vi "RTS Station Save Settings.vi"(8 "Error In":errorcluster, 10 "Data":T1={"Clients"=[], "Listener"=refnum, "Data Array"=["1-1 PF C:\\Technology Lab\\NI-2010\\Trunk\\Refrigeration\\RTS\\Old System\\Point\\16P00290.Pnt"]}, 11 "RTS Config Setup Input":T2) -> (0 "Error Out":errorcluster, 3 "RTS Config Setup Output":T2)   [LabVIEW 2016]
uses:
  Type Definitions/RTS Configuration Setup.ctl
  Type Definitions/RTS Wago Config.ctl
  Type Definitions/RTS APLUS Config.ctl
  Type Definitions/RTS Yokogawa MX Config.ctl
  Type Definitions/RTS Replay Server Control.ctl
  Type Definitions/RTS Server Configuration.ctl
  Type Definitions/RTS Station Settions TCP Comms.ctl
  Type Definitions/RTS Chamber Save Status.ctl
  Type Definitions/RTS Test Pattern.ctl
  Type Definitions/RTS TCP Multiple Connections Data.ctl
  <vilib>/Utility/error.llb/whitespace.ctl
  Type Definitions/RTS TCP Commands.ctl
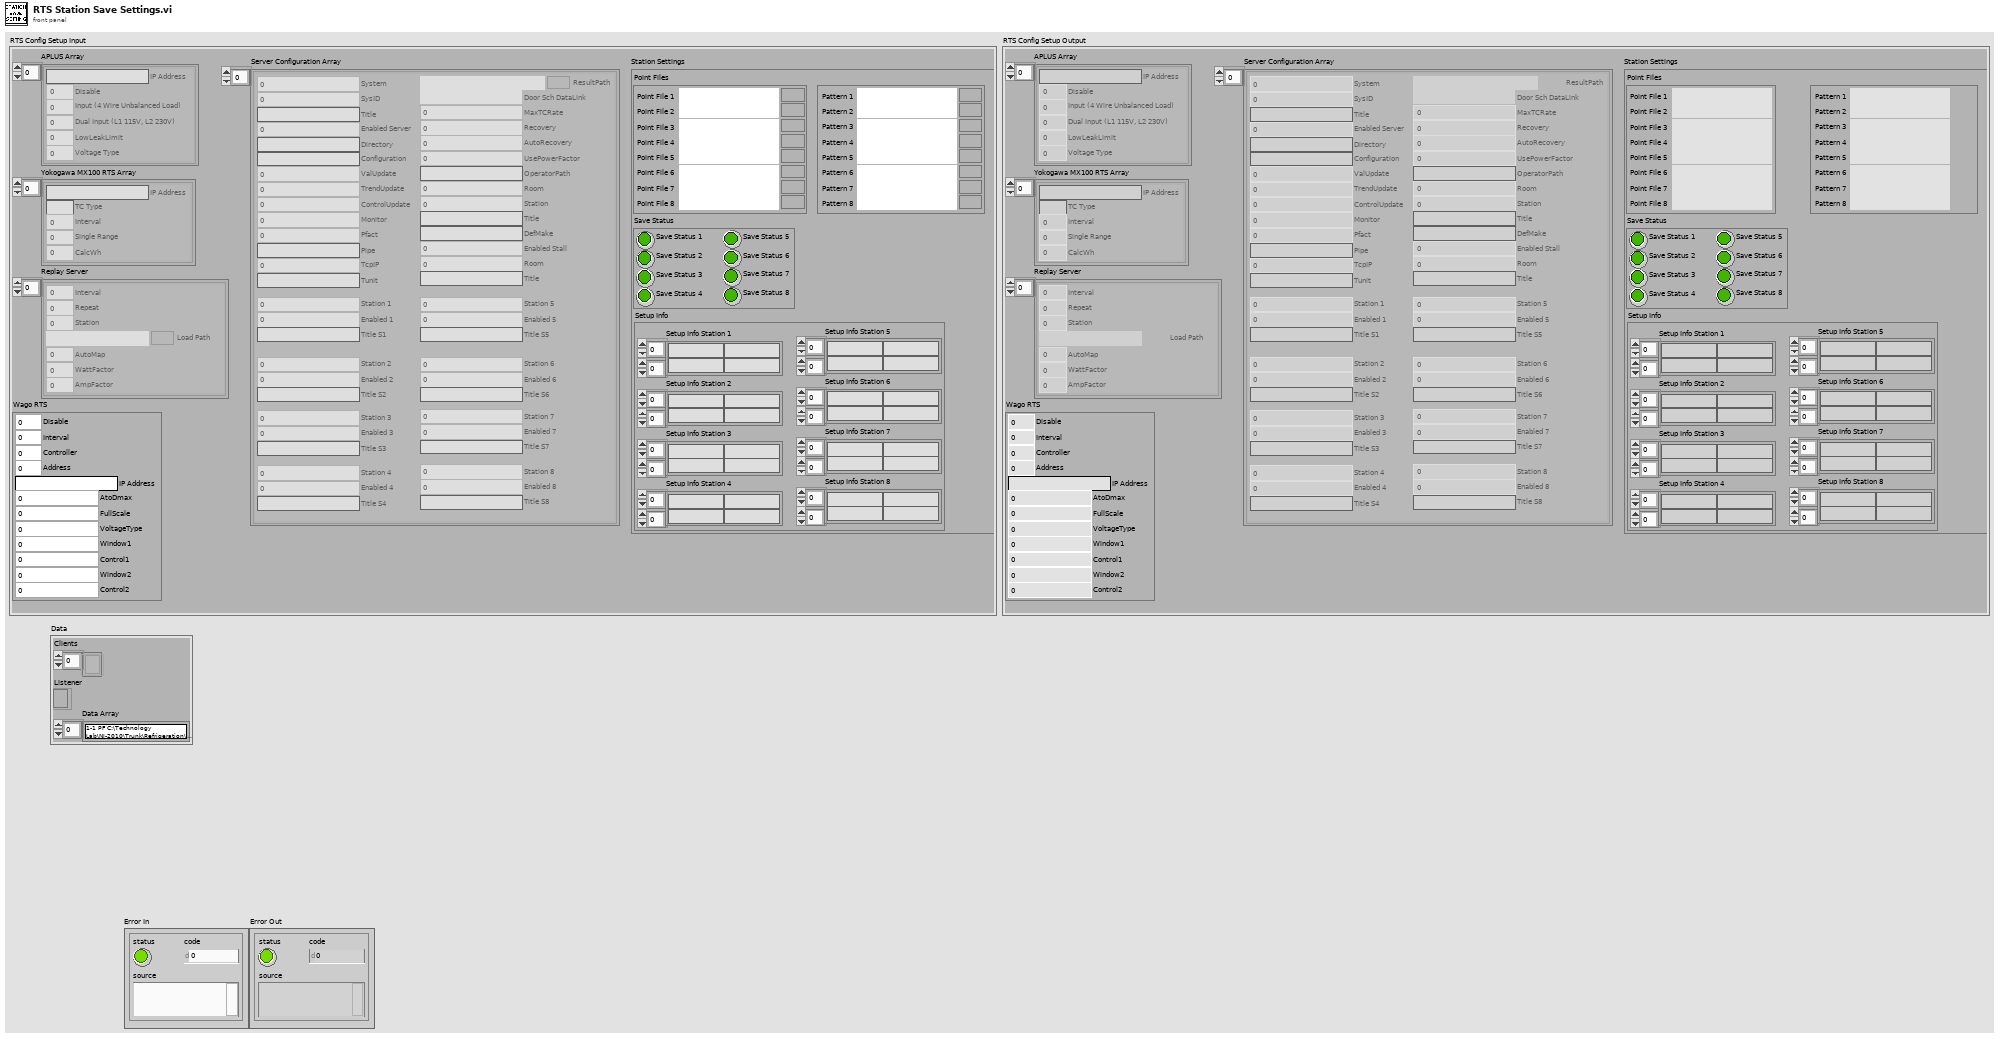
[diagram p1: front panel]
types:
  T1 = typedef "RTS TCP Multiple Connections Data.ctl" = cluster{"Clients":refnum<k5>[], "Listener":refnum<k5>, "Data Array":string[]}
  T2 = typedef "RTS Configuration Setup.ctl" = cluster{"Wago RTS":T3, "APLUS Array":T4[], "Yokogawa MX100 RTS Array":T5[], "Replay Server":T6[], "Server Configuration Array":T7[], "Station Settings":T8}
  T3 = typedef "RTS Wago Config.ctl" = cluster{"Disable":u16, "Interval":u16, "Controller":u16, "Address":u16, "IP Address":string, "AtoDmax":u16, "FullScale":u16, "VoltageType":u16, "Window1":u16, "Control1":u16, "Window2":u16, "Control2":u16}
  T4 = typedef "RTS APLUS Config.ctl" = cluster{"Disable":u16, "IP Address":string, "Input (4 Wire Unbalanced Load)":u16, "Dual Input (L1 115V, L2 230V)":u16, "LowLeakLimit":dbl, "Voltage Type":u16}
  T5 = typedef "RTS Yokogawa MX Config.ctl" = cluster{"IP Address":string, "TC Type":string, "Interval":u16, "Single Range":u16, "CalcWh":u16}
  T6 = typedef "RTS Replay Server Control.ctl" = cluster{"Interval":i16, "Repeat":u16, "Station":u16, "Load Path":path, "AutoMap":u16, "WattFactor":dbl, "AmpFactor":dbl}
  T7 = typedef "RTS Server Configuration.ctl" = cluster{"System":u16, "SysID":u16, "Title":string, "Enabled Server":u16, "Directory":string, "Configuration":string, "ValUpdate":u16, "TrendUpdate":u16, "ControlUpdate":u16, "Monitor":u16, "Pfact":u16, "Pipe":string, "TcpIP":u16, "Tunit":string, "ResultPath":path, "Door Sch DataLink":path, "MaxTCRate":u16, "Recovery":u16, "AutoRecovery":u16, "UsePowerFactor":u16, "OperatorPath":string, "Room":u16, "Station":u16, "Title":string, "DefMake":string, "Enabled Stall":u16, "Room":u16, "Title":string, "Station 1":u16, "Enabled 1":u16, "Station 2":u16, "Enabled 2":u16, "Station 3":u16, "Enabled 3":u16, "Station 4":u16, "Enabled 4":u16, "Station 5":u16, "Enabled 5":u16, "Station 6":u16, "Enabled 6":u16, "Station 7":u16, "Enabled 7":u16, "Station 8":u16, "Enabled 8":u16, "Title S1":string, "Title S2":string, "Title S3":string, "Title S5":string, "Title S6":string, "Title S7":string, "Title S8":string, "Title S4":string}
  T8 = typedef "RTS Station Settions TCP Comms.ctl" = cluster{"Point Files":cluster{"Point File 1":path, "Point File 2":path, "Point File 3":path, "Point File 4":path, "Point File 5":path, "Point File 6":path, "Point File 7":path, "Point File 8":path}, "Save Status":T9, "Setup Info":cluster{"Setup Info Station 1":string[][], "Setup Info Station 2":string[][], "Setup Info Station 3":string[][], "Setup Info Station 4":string[][], "Setup Info Station 5":string[][], "Setup Info Station 6":string[][], "Setup Info Station 7":string[][], "Setup Info Station 8":string[][]}, "Chamber Test Pattern":T10}
  T9 = typedef "RTS Chamber Save Status.ctl" = cluster{"Save Status 1":bool, "Save Status 2":bool, "Save Status 3":bool, "Save Status 4":bool, "Save Status 5":bool, "Save Status 6":bool, "Save Status 7":bool, "Save Status 8":bool}
  T10 = typedef "RTS Test Pattern.ctl" = cluster{" Pattern 1":path, "Pattern 2":path, "Pattern 3":path, "Pattern 4":path, "Pattern 5":path, "Pattern 6":path, "Pattern 7":path, "Pattern 8":path}
  T11 = typedef "RTS TCP Commands.ctl" = string
  T12 = typedef "whitespace.ctl" = u16
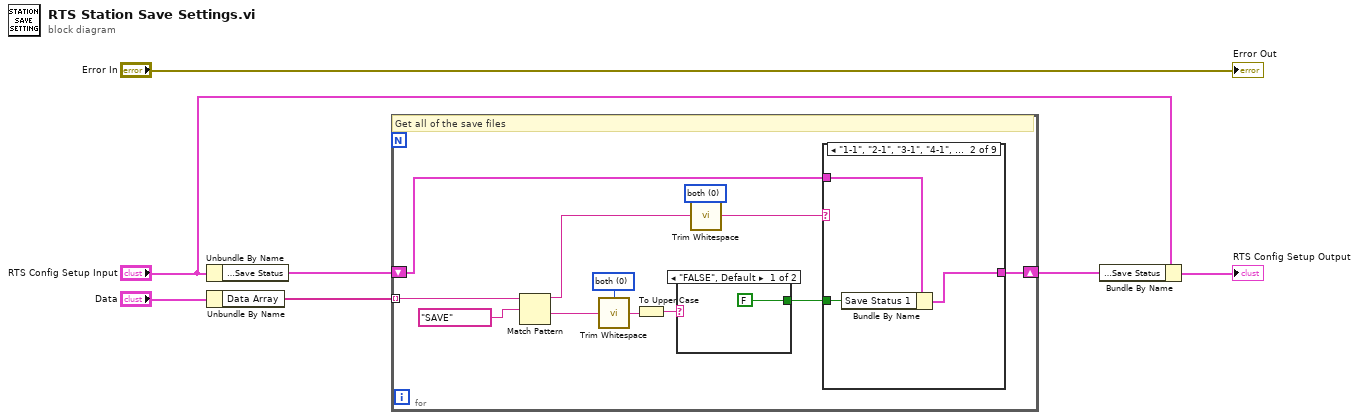
[diagram p0: block diagram]
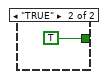
[diagram p2: hidden frame]
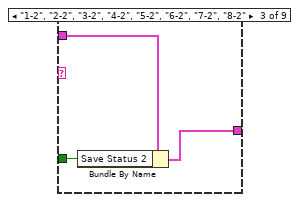
[diagram p4: hidden frame]
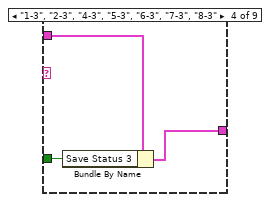
[diagram p5: hidden frame]
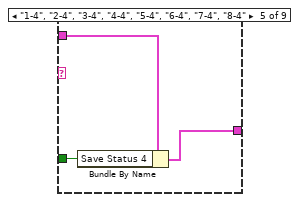
[diagram p6: hidden frame]
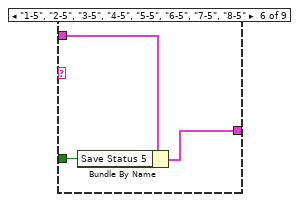
[diagram p7: hidden frame]
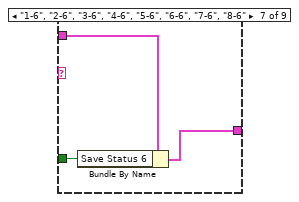
[diagram p8: hidden frame]
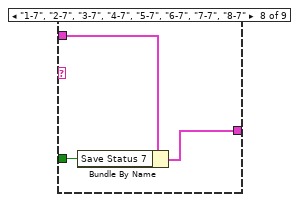
[diagram p9: hidden frame]
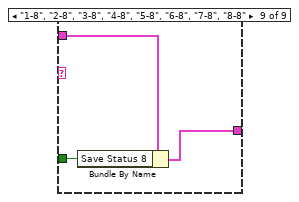
[diagram p10: hidden frame]
diagram:
  n1 = Unbundle By Name("RTS Config Setup Input") -> ("Station Settings.Save Status"=w4:T9)
  n2 = Unbundle By Name("Data") -> ("Data Array"=w6:string[])
  n3 = for {
    tunnel: w6 -> [w18] mode=indexing
    shift-right: [w13] -> w1
    shift-left: w4 -> [w14]
    w9 = T12 0 items=["both", "start of string", "end of string"] ("location (both)")
    w19 = T12 0 items=["both", "start of string", "end of string"] ("location (both)")
    # "Get all of the save files"
    n4 = Match Pattern(string=w18, regular expression=T11 "SAVE" ("TCP Commands")) -> (before substring=w17:string, after substring=w16:string)  [unwired: 1 in, 2 out]
    n5 = call <vilib>:"Trim Whitespace.vi"("string"=w16, "location (both)"=w19) -> ("trimmed string"=w12:string)
    n6 = To Upper Case(1:w12) -> (0:w11:string)
    n7 = case shown="\"FALSE\", Default" w11 {
      tunnel: [FALSE TRUE] -> w10
      frame "FALSE", Default {
      }
      frame "TRUE" {
      }
    }
    n8 = call <vilib>:"Trim Whitespace.vi"("string"=w17, "location (both)"=w9) -> ("trimmed string"=w15:string)
    n9 = case shown="\"1-1\", \"2-1\", \"3-1\", \"4-1\", \"5-1\", \"6-1\", \"7-1\", \"8-1\"" w15 {
      tunnel: w14 -> [w22 w25 w28 w31 w34 w37 w40 w43 w46]
      tunnel: [w22 w24 w27 w30 w33 w36 w39 w42 w45] -> w13
      tunnel: w10 -> [_ w23 w26 w29 w32 w35 w38 w41 w44]
      frame Default {
      }
      frame "1-1", "2-1", "3-1", "4-1", "5-1", "6-1", "7-1", "8-1" {
        n10 = Bundle By Name(cluster=w25, "Save Status 1"=w23) -> (w24:T9)
      }
      frame "1-2", "2-2", "3-2", "4-2", "5-2", "6-2", "7-2", "8-2" {
        n11 = Bundle By Name(cluster=w28, "Save Status 2"=w26) -> (w27:T9)
      }
      frame "1-3", "2-3", "4-3", "5-3", "6-3", "7-3", "8-3" {
        n12 = Bundle By Name(cluster=w31, "Save Status 3"=w29) -> (w30:T9)
      }
      frame "1-4", "2-4", "3-4", "4-4", "5-4", "6-4", "7-4", "8-4" {
        n13 = Bundle By Name(cluster=w34, "Save Status 4"=w32) -> (w33:T9)
      }
      frame "1-5", "2-5", "3-5", "4-5", "5-5", "6-5", "7-5", "8-5" {
        n14 = Bundle By Name(cluster=w37, "Save Status 5"=w35) -> (w36:T9)
      }
      frame "1-6", "2-6", "3-6", "4-6", "5-6", "6-6", "7-6", "8-6" {
        n15 = Bundle By Name(cluster=w40, "Save Status 6"=w38) -> (w39:T9)
      }
      frame "1-7", "2-7", "3-7", "4-7", "5-7", "6-7", "7-7", "8-7" {
        n16 = Bundle By Name(cluster=w43, "Save Status 7"=w41) -> (w42:T9)
      }
      frame "1-8", "2-8", "3-8", "4-8", "5-8", "6-8", "7-8", "8-8" {
        n17 = Bundle By Name(cluster=w46, "Save Status 8"=w44) -> (w45:T9)
      }
    }
  }
  n18 = Bundle By Name(cluster="RTS Config Setup Input", "Station Settings.Save Status"=w1) -> (→"RTS Config Setup Output":T2)
  "Error Out" <- "Error In"
